vi "CoboltLaser_OperatingHoursGet.vi"(0 "ComPort":refnum<visa-resource-name>, 3 "GenerateError":bool=TRUE, 7 "error in (no error)":errorcluster) -> (20 "ComPortOut":refnum<visa-resource-name>, 21 "OperatingHours":dbl, 27 "error out":errorcluster)   [LabVIEW 2019]
doc: "Use this template to build a VI to use as a subVI."
uses:
  <userlib>/CoboltLaser/CoboltLaser_Controls/ExpectedResponseType.ctl
panel:
  out "ResponseOK":bool
  out "Response":string
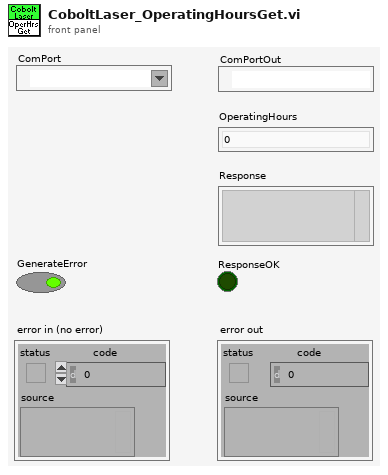
[diagram p1: front panel]
types:
  T1 = typedef "ExpectedResponseType.ctl" = enum16{"Any", "Digits Only", "Non-Digits Only"}
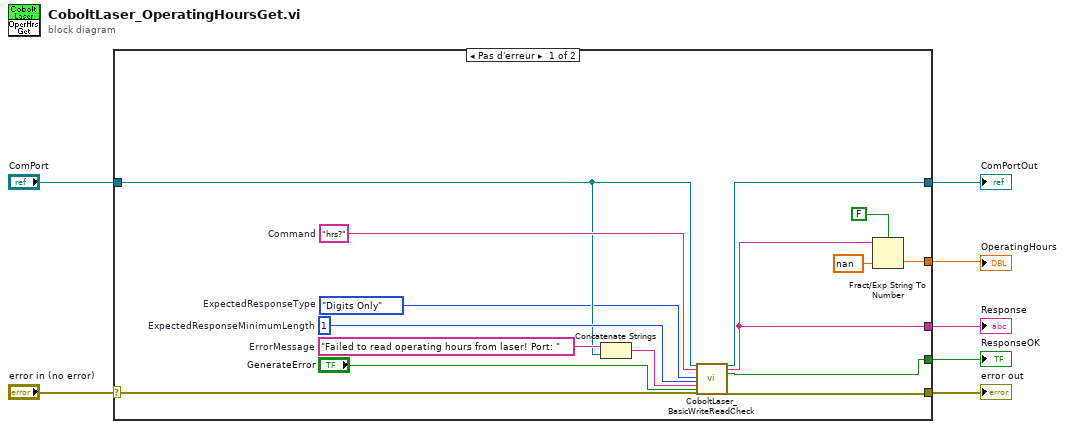
[diagram p0: block diagram]
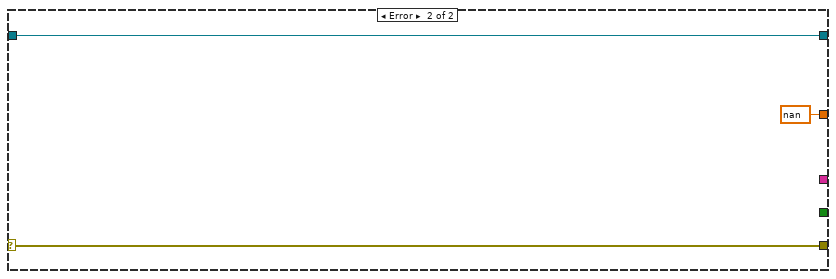
[diagram p2: hidden frame]
diagram:
  n1 = case shown="Pas d'erreur" "error in (no error)" {
    selector: "error in (no error)" -> [w22 w25]
    tunnel: [w21 w25] -> w6
    tunnel: "ComPort" -> [w15 w24]
    tunnel: [w14 w24] -> w4
    tunnel: [w10 nan] -> w3
    tunnel: [w9 _] -> w2
    tunnel: [w8 _] -> w1
    frame No Error {
      w12 = ExpectedResponseType."Digits Only"  # ExpectedResponseType
      w19 = 1  # ExpectedResponseMinimumLength
      w17 = "Failed to read operating hours from laser! Port: "  # ErrorMessage
      w20 = "hrs?"  # Command
      n2 = Concatenate Strings(w17, w15) -> (w16:string)
      n3 = call <userlib>:"CoboltLaser_BasicWriteReadCheck.vi"("ComPort"=w15, "Command"=w20, "ExpectedResponseType"=w12, "ExpectedResponseMinimumLength"=w19, "ErrorMessage"=w16, "GenerateError"="GenerateError", "error in (no error)"=w22) -> ("ComPortOut"=w14:refnum<visa-resource-name>, "Response"=w8:string, "ResponseOK"=w9:bool, "error out"=w21:errorcluster)  [unwired: 17 in]
      n4 = Fract/Exp String To Number(use system decimal point (T)=FALSE, string=w8, default (0 dbl)=nan ("default (0 DBL)")) -> (number=w10:dbl)  [unwired: 1 in, 1 out]
    }
    frame Error {
    }
  }
  "error out" <- w6
  "ComPortOut" <- w4
  "Response" <- w1
  "ResponseOK" <- w2
  "OperatingHours" <- w3
